vi "RumbleControl.vi"(10 "Teleop Time":dbl, 11 "JoystickDevRef":T1) -> ()   [LabVIEW 2016]
uses:
  <vilib>/Rock Robotics/WPI/Joystick/WPI_JoystickDevRef.ctl
  <vilib>/Rock Robotics/WPI/Joystick/WPI_JoystickDeviceEnum.ctl
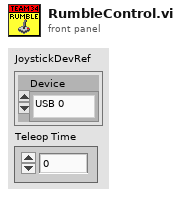
[diagram p1: front panel]
types:
  T1 = typedef "WPI_JoystickDevRef.ctl" = cluster{"Device":T2}
  T2 = typedef "WPI_JoystickDeviceEnum.ctl" = enum16{"USB 0", "USB 1", "USB 2", "USB 3", "USB 4", "USB 5"}
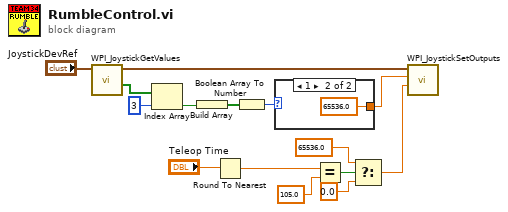
[diagram p0: block diagram]
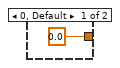
[diagram p2: hidden frame]
diagram:
  n1 = call <vilib>:"WPI_JoystickGetValues.vi"("JoystickDevRef"="JoystickDevRef") -> ("Buttons"=w14:bool[], "JoystickDevRef"=w7:T1)  [unwired: 6 in, 3 out]
  n2 = Index Array(array=w14, index=3) -> (element=w12:bool)
  n3 = Build Array(w12) -> (w11:bool[])
  n4 = Round To Nearest(number="Teleop Time") -> (nearest integer value=w5:dbl)
  n5 = Boolean Array To Number(Boolean array=w11) -> (number=w10:u32)
  n6 = case shown="1" w10 {
    tunnel: [sgl 0.0 ("Left Rumble") sgl 65536.0 ("Left Rumble")] -> w9
    frame 0, Default {
    }
    frame 1 {
    }
  }
  n7 = Equal?(x=w5, y=105.0) -> (x = y?=w4:bool)
  n8 = Select(t=sgl 65536.0 ("Left Rumble"), s=w4, f=sgl 0.0) -> (s? t:f=w1:sgl)
  n9 = call <vilib>:"WPI_JoystickSetOutputs.vi"("Right Rumble"=w1, "Left Rumble"=w9, "JoystickDevRef"=w7) -> ()  [unwired: 7 in, 2 out]
